vi "Pic Overlay b Box.vi"(8 "error in (no error)":errorcluster, 11 "LF2R IDE in":refnum<class "Main Panel.lvclass">) -> (0 "error out":errorcluster, 3 "LF2R IDE out":refnum<class "Main Panel.lvclass">)   [LabVIEW 2018, in "Main Panel.lvlib" / "Main Panel.lvclass"]
uses:
  Main Panel.lvclass
  Main Panel.lvclass/Main Panel.ctl
  Picture Process/Picture Process.lvclass
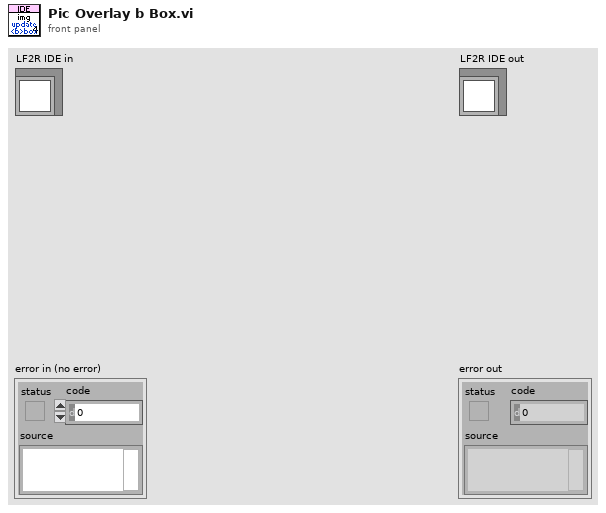
[diagram p1: front panel]
types:
  T1 = typedef "Data Parser.lvclass/frame b data.ctl" = cluster{"kind":string, "x":string, "y":string, "w":string, "h":string}
  T2 = cluster{"Fill Color":u32, "Border Color":u32, "Show?":bool}
  T3 = cluster{"x":string, "y":string, "w":string, "h":string}
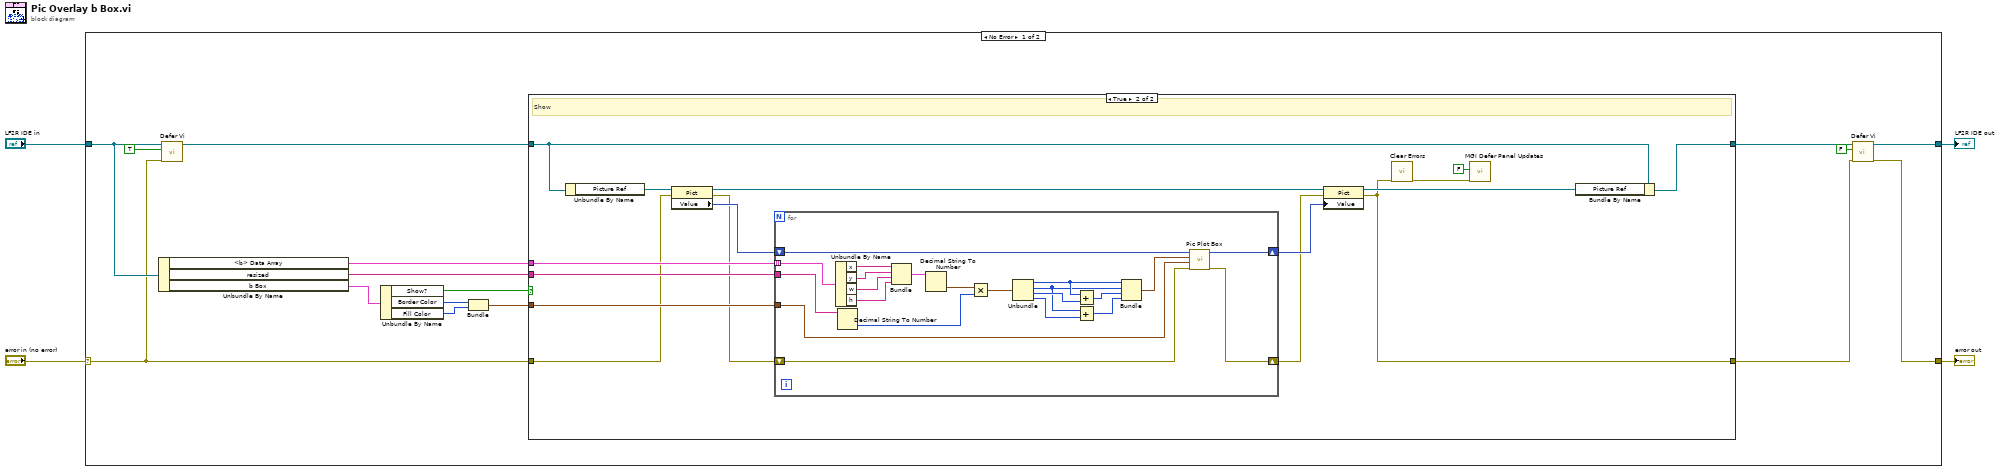
[diagram p0: block diagram]
diagram:
  n1 = case shown="No Error" "error in (no error)" {
    selector: "error in (no error)" -> [w12 w62]
    tunnel: [w7 w62] -> w3
    tunnel: [w9 w61] -> w1
    tunnel: "LF2R IDE in" -> [w13 w61]
    frame No Error {
      n2 = Unbundle By Name(w13) -> ("<b> Data Array"=w20:T1[], "resized"=w19:string, "b Box"=w18:T2)
      n3 = call "Defer Vi.vi"("error in (no error)"=w12, "Defer Updates?"=TRUE, "Main Panel in"=w13) -> ("Main Panel out"=w11:refnum<class "Main Panel.lvclass">)  [unwired: 7 in, 1 out]
      n4 = Unbundle By Name(w18) -> ("Show?"=w17:bool, "Border Color"=w16:u32, "Fill Color"=w15:u32)
      n5 = Bundle("Border Color"=w16, "Fill Color"=w15) -> (w14:cluster{"Border Color":u32, "Fill Color":u32})  [unwired: 1 in]
      n6 = case shown="True" w17 {
        tunnel: w20 -> [_ w38]
        tunnel: w12 -> [w21 w33]
        tunnel: w11 -> [w22 w23]
        tunnel: [w21 w26] -> w8
        tunnel: w19 -> [_ w37]
        tunnel: [w22 w29] -> w10
        tunnel: w14 -> [_ w36]
        frame False {
          # "Skip"
        }
        frame True {
          # "Show"
          n7 = Unbundle By Name(w23) -> ("Picture Ref"=w35:refnum<vi>)
          n8 = property class="Pict"(reference=w35, error in=w33) -> (reference out=w32:refnum<vi>, error out=w27:errorcluster, "Value"=w34:picture)
          n9 = for {
            tunnel: w38 -> [w60] mode=indexing
            shift-right: [w40] -> w30
            shift-left: w27 -> [w41]
            shift-right: [w39] -> w31
            shift-left: w34 -> [w44]
            tunnel: w37 -> [w46]
            tunnel: w36 -> [w42]
            n10 = Unbundle By Name(w60) -> ("x"=w57:string, "y"=w56:string, "w"=w55:string, "h"=w54:string)
            n11 = Decimal String To Number(string=w46) -> (number=w45:i32)  [unwired: 2 in, 1 out]
            n12 = Bundle("x"=w57, "y"=w56, "w"=w55, "h"=w54) -> (w53:T3)  [unwired: 1 in]
            n13 = Decimal String To Number(string=w53) -> (number=w48:cluster{"x":i32, "y":i32, "w":i32, "h":i32})  [unwired: 2 in, 1 out]
            n14 = Multiply(x=w48, y=w45) -> (x*y=w47:cluster{"x":i32, "y":i32, "w":i32, "h":i32})
            n15 = Unbundle(w47) -> ("x"=w52:i32, "y"=w50:i32, "w"=w51:i32, "h"=w49:i32)
            n16 = Add(x=w52, y=w51) -> (x+y=w59:i32)
            n17 = Add(x=w50, y=w49) -> (x+y=w58:i32)
            n18 = Bundle("x"=w52, "y"=w50, w59, w58) -> (w43:cluster{"x":i32, "y":i32, i32, i32})  [unwired: 1 in]
            n19 = call "Pic Plot Box.vi"("error in (no error)"=w41, "Color"=w42, "Rectangle"=w43, "Picture in"=w44) -> ("error out"=w40:errorcluster, "Picture out"=w39:picture)  [unwired: 6 in]
          }
          n20 = property class="Pict"(reference=w32, error in=w30, "Value"=w31) -> (reference out=w28:refnum<vi>, error out=w26:errorcluster)
          n21 = call <vilib>:"Clear Errors.vi"("error in (no error)"=w26) -> ("error out"=w25:errorcluster)  [unwired: 5 in, 1 out]
          n22 = call <userlib>:"MGI Defer Panel Updates.vi"("Error In"=w25, "Defer Updates?"=FALSE) -> ()  [unwired: 9 in, 1 out]
          n23 = Bundle By Name(cluster=w23, "Picture Ref"=w28) -> (w29:refnum<class "Main Panel.lvclass">)
        }
      }
      n24 = call "Defer Vi.vi"("error in (no error)"=w8, "Defer Updates?"=FALSE, "Main Panel in"=w10) -> ("error out"=w7:errorcluster, "Main Panel out"=w9:refnum<class "Main Panel.lvclass">)  [unwired: 7 in]
    }
    frame Error {
    }
  }
  "error out" <- w3
  "LF2R IDE out" <- w1
